vi "IdentityCheck.vi"(8 "error in (no error)":errorcluster, 11 "CEG4500 in":refnum<class "CEG4500.lvclass">) -> (0 "error out":errorcluster, 3 "CEG4500 out":refnum<class "CEG4500.lvclass">)   [LabVIEW 2013, in "CEG4500.lvclass"]
uses:
  CEG4500.lvclass
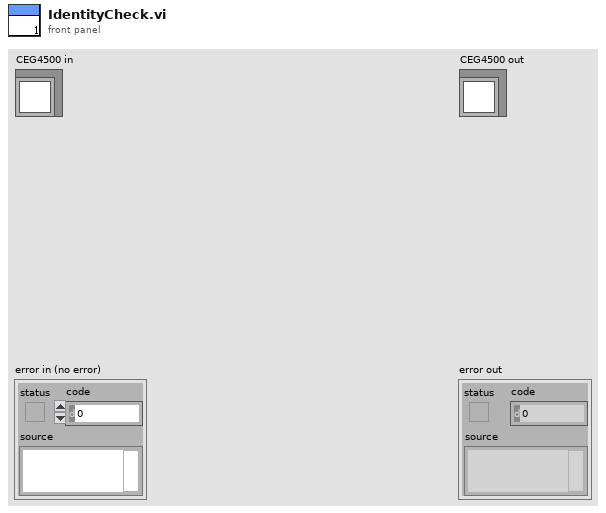
[diagram p1: front panel]
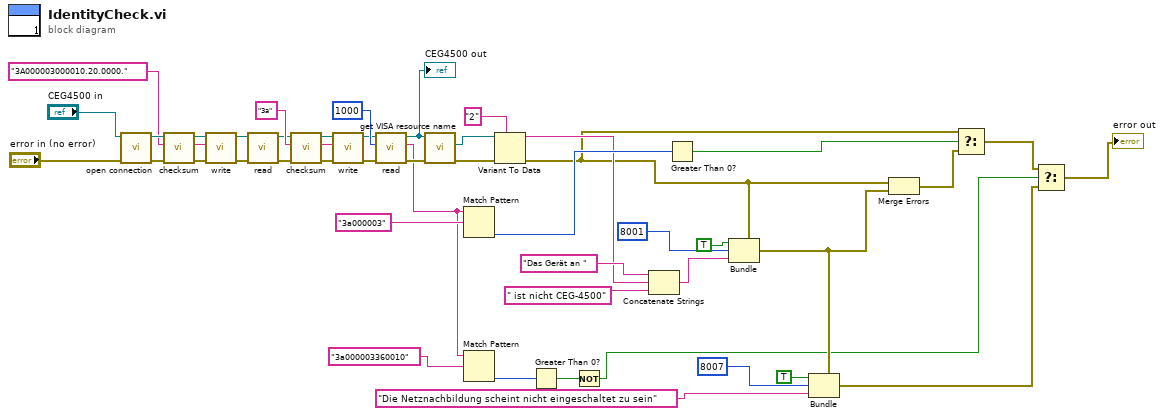
[diagram p0: block diagram]
diagram:
  n1 = call-dynamic "open connection.vi"("error in (no error)"="error in (no error)", "CEG4500 in"="CEG4500 in") -> ("error out"=w45:errorcluster, "CEG4500 out"=w46:refnum<class "CEG4500.lvclass">)  [unwired: 8 in]
  n2 = call-dynamic "checksum.vi"("error in (no error)"=w45, "input"="3A000003000010.20.0000.", "CEG4500 in"=w46) -> ("error out"=w44:errorcluster, "output"=w41:string, "CEG4500 out"=w43:refnum<class "CEG4500.lvclass">)  [unwired: 6 in]
  n3 = call-dynamic "write.vi"("error in (no error)"=w44, "String to send"=w41, "CEG4500 in"=w43) -> ("error out"=w19:errorcluster, "CEG4500 out"=w20:refnum<class "CEG4500.lvclass">)  [unwired: 7 in]
  n4 = call-dynamic "read.vi"("error in (no error)"=w19, "CEG4500 in"=w20) -> ("error out"=w18:errorcluster, "CEG4500 out"=w17:refnum<class "CEG4500.lvclass">)  [unwired: 7 in, 1 out]
  n5 = call-dynamic "checksum.vi"("error in (no error)"=w18, "input"="3a", "CEG4500 in"=w17) -> ("error out"=w26:errorcluster, "output"=w24:string, "CEG4500 out"=w23:refnum<class "CEG4500.lvclass">)  [unwired: 6 in]
  n6 = call-dynamic "write.vi"("error in (no error)"=w26, "String to send"=w24, "CEG4500 in"=w23) -> ("error out"=w22:errorcluster, "CEG4500 out"=w16:refnum<class "CEG4500.lvclass">)  [unwired: 7 in]
  n7 = call-dynamic "read.vi"("error in (no error)"=w22, "timeout (ms)"=1000, "CEG4500 in"=w16) -> ("error out"=w21:errorcluster, "Return String"=w11:string, "CEG4500 out"=w15:refnum<class "CEG4500.lvclass">)  [unwired: 6 in]
  "CEG4500 out" <- w15
  n8 = call-dynamic "get VISA resource name.vi"("error in (no error)"=w21, "DeviceInterface (Eingang)"=w15) -> ("error out"=w14:errorcluster, "VISA resource name"=w36:refnum<visa-resource-name>)  [unwired: 7 in, 1 out]
  n9 = Match Pattern(string=w11, regular expression="3a000003") -> (offset past match=w38:i32)  [unwired: 1 in, 3 out]
  n10 = Match Pattern(string=w11, regular expression="3a000003360010") -> (offset past match=w10:i32)  [unwired: 1 in, 3 out]
  n11 = Variant To Data(error in=w14, type="2" ("input"), Variant=w36) -> (data=w30:string, error out=w13:errorcluster)
  n12 = Greater Than 0?(x=w10) -> (x > 0?=w3:bool)
  n13 = Not(x=w3) -> (.not. x?=w2:bool)
  n14 = Concatenate Strings("Das Gerät an " ("string"), w30, " ist nicht CEG-4500" ("string")) -> (w28:string)
  n15 = Greater Than 0?(x=w38) -> (x > 0?=w37:bool)
  n16 = Bundle(cluster=w13, "status"=TRUE, "code"=8001, "source"=w28) -> (w6:errorcluster)
  n17 = Bundle(cluster=w6, "status"=TRUE, "code"=8007, "source"="Die Netznachbildung scheint nicht eingeschaltet zu sein" ("string")) -> (w4:errorcluster)
  n18 = Merge Errors(w13, w6) -> (w27:errorcluster)
  n19 = Select(t=w13, s=w37, f=w27) -> (s? t:f=w5:errorcluster)
  n20 = Select(t=w5, s=w2, f=w4) -> (s? t:f=→"error out":errorcluster)
